vi "PI Terminal.vi"() -> ()   [LabVIEW 2013]
doc: "HELP for Terminal.vi\n\nThe terminal VI is a stand-alone application. It first asks the user to specify the full configuration (number of controlled systems, RS-232, GPIB, TCP-IP or DLL communication, communications parameters), then it establishes a connection with a selected system. This will work for all PI devices which support the PI General Command Set, or at least follow the same syntax rules and support the *IDN? and ERR? commands.\n\nAfter starting the VI, the interface parameters of the systems with which to communicate must be selected. For this reason, \"PITerminal.vi\" calls \"PI Ask for Communication Parameters.vi\". Select here the number of connected PI systems that you want to communicate with. For each system, select the appropriate interface parameters. \n\nC-702: Interface = RS232 or TCP/IP, RS232: Input and output HW handshake must be TRUE. Syntax: GCS 1.0; Term char = LF.\n\nC-843: Interface = DLL, DLL for Device = C-843, DLL Interface = Board, Parameter = Board number (1 for first C-843 board). Syntax: GCS 1.0; Term char = LF.\n\nC-843.PM: Interface = DLL, DLL for Device = C-843.PM, DLL Interface = Board, Parameter = Board number (1 for first C-843 board). Syntax: GCS 1.0; Term char = LF.\n\nC-844: Interface = DLL, DLL for Device = C-844, DLL Interface = RS232 or GPIB, Parameter = empty string, RS232 baud rate = 9600. Syntax: GCS 1.0; Term char = LF.\n\nC-865: Interface = DLL, DLL for Device = C-865, DLL Interface = RS232, Parameter = empty string, RS232 baud rate = set as appropriate. Syntax: GCS 1.0; Term char = LF.\n\nC-866: Interface = DLL, DLL for Device = C-866, DLL Interface = RS232 or USB, RS232: Parameter = empty string, RS232 baud rate = set as appropriate, USB: Parameter = Serial no. of system to connect to, Syntax: GCS 1.0; Term char = LF.\n\nC-867: Single Device: Interface = RS232 or DLL, RS232: Input and output HW handshake must be FALSE. DLL (USB): DLL for Device = C-867, DLL Interface = USB, Parameter = Serial no. of system to connect to. DaisyChain: Interface = DLL, DLL for Device = C-867, DLL Interface = RS232_DC, Parameter = Number of device in chain, Register DC: FALSE. Syntax: GCS 2.0; Term char = LF.\n\nC-880, C-848: Interface = RS232 or GPIB, RS232: Input and output HW handshake must be TRUE. Syntax: GCS 1.0; Term char = LF.\n\nC-880K005: Interface = RS232, Input and output HW handshake must be FALSE. Syntax: GCS 1.0; Term char = LF.\n\nE-516: Interface = RS232 or GPIB, RS232: Input and output HW handshake must be TRUE. Syntax: GCS 1.0; Term char = LF.\n\nE-517: Interface = RS232, GPIB, TCP/IP or DLL, RS232: Input and output HW handshake must be TRUE, DLL (USB): DLL for Device = E-517, DLL Interface = USB, Parameter = Serial no. of system to connect to. Syntax: GCS 2.0; Term char = LF.\n\nE-709: Interface = RS232 or DLL, RS232: Input and output HW handshake must be TRUE. DLL (USB): DLL for Device = E-709, DLL Interface = USB, Parameter = Serial no. of system to connect to. Syntax: GCS 2.0; Term char = LF.\n\nE-710: Interface = DLL, DLL for Device = E-710, DLL Interface = RS232 or GPIB, Parameter = empty string. Syntax: GCS 1.0; Term char = LF.\n\nE-712: Interface = RS232, TCP/IP or DLL, RS232: Input and output HW handshake must be TRUE. DLL: DLL for Device = E-712, DLL Interface = USB, Parameter = Serial no. of system to connect to. Syntax: GCS 2.0; Term char = LF.\n\nE-725: Interface = RS232, TCP/IP or DLL, RS232: Input and output HW handshake must be TRUE. DLL: DLL for Device = E-725, DLL Interface = USB, Parameter = Serial no. of system to connect to. Syntax: GCS 2.0; Term char = LF.\n\nE-753: Interface = RS232 or TCP/IP, RS232: Input and output HW handshake must be TRUE. Syntax: GCS 2.0; Term char = LF.\n\nE-755: Single Device: Interface = RS232, Input and output HW handshake must be TRUE. DaisyChain: Interface = DLL, DLL for Device = E-755, DLL Interface = RS232_DC, Parameter = Number of device in chain (first device: 1). Syntax: GCS 2.0; Term char = LF.\n\nE-761: Interface = DLL, DLL for Device = E-761, DLL Interface = Board, Parameter = Board number (1 for first E-761 board). Syntax: GCS 1.0; Term char = LF.\n\nE-816: Interface = RS232 or DLL, RS232: Input and output HW handshake must be TRUE. DLL (USB): DLL for Device = E-816, DLL Interface = USB, Parameter = Serial no. of system to connect to. Syntax: GCS 1.0; Term char = LF. \n\nE-861: Single Device: Interface = RS232 or DLL, RS232: Input and output HW handshake must be FALSE. DLL (USB): DLL for Device = E-861, DLL Interface = USB, Parameter = Serial no. of system to connect to. DaisyChain: Interface = DLL, DLL for Device = E-861, DLL Interface = RS232_DC, Parameter = Number of device in chain (first device: 1), Register DC: FALSE. Syntax: GCS 2.0; Term char = LF.\n\nF-206, M-8X0: For GCS syntax version = GCS 1.0 (older firmware or compatibility mode, can be set with CSV.vi), Interface = RS232, GPIB (not available for C-887 controller) or TCP/IP., The error status will not be cleared by this VI. The first ERR? query will report a hidden error with error code 1, which will be cleared during system initialization (INI). RS232: Input and output handshake settings must be FALSE. Syntax: GCS 1.0; Term char = LF.\n For GCS syntax version = GCS 2.0 (C-887 Controller), Interface = RS232 or TCP/IP. RS232: Input and output handshake settings must be FALSE. Syntax: GCS 2.0; Term char = LF.\n\nMercury™: Interface = DLL, DLL for Device = Mercury™, DLL Interface = RS232 (even if using USB), Parameter = empty string, RS232 baud rate = same as set on controller hardware. Syntax: GCS 1.0; Term char = LF.\n\nGCS_Mercury: Single Device: Interface = RS232 or DLL, RS232: Input and output HW handshake must be FALSE. DLL (USB): DLL for Device = PI_GCS2_DLL, DLL Interface = USB, Parameter = Serial no. of system to connect to.\n DaisyChain: Interface = DLL, DLL for Device = PI_GCS2_DLL, DLL Interface = RS232_DC, Parameter = Number of device in chain, Register DC: FALSE. Syntax: GCS 2.0; Term char = LF.\n\nIf the chosen timeout value is greater than 1000 ms, it will automatically be set to 1000 ms for a fluid program operation. \n\nIn the upper window (\"Send\") the user can enter commands which will be transmitted to the chosen device one line at a time when the ENTER key is pressed. \nAll controller responses are displayed in the Receive response window, which can be cleared by pressing the Clear Receive Window button or F2. \n\nThe view style of the Receive window can be changed to Show all characters or Hex View using the menu ring above the Receive window.\n\nExit or F10 will terminate the terminal application. \n\nTo send the last command again, just press the ENTER key again. The next line will then show the following entry: \"(Send: cmd)\" with cmd being the command from the line before, which was resent.\n\nWhen the terminal application has just been started, pressing ENTER without entering a command will send \"*IDN?\" to the chosen system. \n\nNew commands can only be inserted into the last line of the Send window. The user can scroll through the history of the Send window using the scroll bar or the cursor up/down keys, but cannot change the history or resend commands by pressing ENTER unless in the last line. Pressing ENTER will always resend the last command, no matter where the cursor is positioned. Selecting text and using copy and paste (Ctrl+C, Ctrl+V) works for single lines, if only the contents of one single line (the command text) is selected and copied, not the full line (including the LineFeed) or multiple lines.\n\nMany of PI's General Command Set compatible devices support single-byte commands. For example, the user can stop a fast scan of a C-880 or F-206 by sending an ASCII 24 (decimal). To enter this command into the Send window simply type a \"#\" followed by the decimal value of the byte to be sent, e.g. enter \"#24\" and presses ENTER to stop a fast scan. An entry \"(Send: *)\" will be added to the original command with * being the corresponding ASCII character of the single byte sent. \n\nPressing F1 or the Help button will pop up a help window. To return to the terminal application, press Esc. If Send ERR? on Exit? is TRUE, an \"ERR?\" query is sent to the device when Exit is pressed to prevent the controller from keeping an error condition produced during the use of the terminal application."
uses:
  Low Level/Communication.llb/Available DLLs.ctl
  Low Level/Communication.llb/Termination character.ctl
panel:
  in  "HowTo":string="Start application and choose interface parameters in next window."
  out "TCP/IP Config. System":T1={"Host address/name"="Z-A521-2.pi.ws", "Port"=3000, "Board"=0, "Timeout"=5000}
  out "Help string":string="\nHELP for Terminal.vi\n\nThis terminal application works for all PI devices which support the PI General Command Set or at least follow the syntax rules of this command structure and support the commands *IDN? and ERR?.\n\nIn the upper window (\"Send\") the user can enter commands which will be transmitted to the chosen device one line at a time when the ENTER key is pressed. All controller responses are displayed in the Receive response window, which can be cleared by pressing the Clear Receive Window button or F2. The view style of the Receive window can be changed to Show all characters or Hex View using the menu ring above the Receive window.\n\nExit or F10 will terminate the terminal application. \n\nTo send the last command again, just press the ENTER key again. The next line will then show the following entry: \"(Send: cmd)\" with cmd being the command from the line before, which was resent.\nWhen the terminal application has just been started, pressing ENTER without entering a command will send \"*IDN?\" to the chosen system.\n\nNew commands can only be inserted into the last line of the Send window. The user can scroll through the history of the Send window using the scroll bar or the cursor up/down keys, but cannot change the history or resend commands by pressing ENTER unless in the last line. Pressing ENTER will always resend the last command, no matter where the cursor is positioned. Selecting text and using copy and paste (Ctrl+C, Ctrl+V) works for single lines, if only the contents of one single line (the command text) is selected and copied, not the full line (including the LineFeed) or multiple lines.\n\nMany of PI's General Command Set compatible devices support single-byte commands. For example, the user can stop a fast scan of a C-880 or F-206 by sending an ASCII 24 (decimal). To enter this command into the Send window simply type a \"#\" followed by the decimal value of the byte to be sent, e.g. enter \"#24\" and presses ENTER to stop a fast scan. An entry \"(Send: *)\" will be added to the original command with * being the corresponding ASCII character of the single byte sent. \n\nIf Send ERR? on Exit? is TRUE, a \"ERR?\" query is sent to the device when Exit is pressed to prevent the controller from keeping an error condition produced during the use of the terminal application.\n\nC-702: \tInterface = RS232 or TCP/IP, RS232: Input and output HW handshake \tmust \tbe TRUE. Syntax: GCS 1.0; Term char = LF.\n\nC-843: \tInterface = DLL, DLL for Device = C-843, DLL Interface = Board, \tParameter = Board number (1 for first C-843 board). Syntax: GCS 1.0; \tTerm char = LF.\n\nC-843.PM: \tInterface = DLL, DLL for Device = C-843.PM, DLL Interface = Board, \tParameter = Board number (1 for first C-843 board). Syntax: GCS 1.0; \tTerm char = LF.\n\nC-865: \tInterface = DLL, DLL for Device = C-865, DLL Interface = RS232, \tParameter = empty string, RS232 baud rate = set as appropriate. Syntax: \tGCS 1.0; Term char = LF.\n\nC-866: \tInterface = DLL, DLL for Device = C-866, DLL Interface = RS232 or USB, \tRS232: Parameter = empty string, RS232 baud rate = set as appropriate, \tUSB: Parameter = Serial no. of system to connect to, \n\tSyntax: GCS 1.0; Term char = LF.\n\nC-867: \tSingle Device: Interface = RS232 or DLL, RS232: Input and output HW \thandshake must be FALSE. DLL (USB): DLL for Device = C-867, DLL \tInterface = USB, Parameter = Serial no. of system to connect to.\nDaisyChain: Interface = DLL, DLL for Device = C-867, DLL Interface = \tRS232_DC, Parameter = Number of device in chain, \tRegister DC: \tFALSE. Syntax: GCS 2.0; Term char = LF.\n\nC-880, C-848: \tInterface = RS232 or GPIB, RS232: Input and output HW handshake must \tbe TRUE. Syntax: GCS 1.0; Term char = LF.\n\nC-880K005: \tInterface = RS232, Input and output HW handshake must be FALSE. \tSyntax: GCS 1.0; Term char = LF.\n\nE-516: \tInterface = RS232 or GPIB, RS232: Input and output HW handshake must \tbe TRUE. Syntax: GCS 1.0; Term char = LF.\n\nE-517: \tInterface = RS232, GPIB, TCP/IP or DLL, RS232: Input and output HW \thandshake must be TRUE, DLL (USB): DLL for Device = E-517, DLL \tInterface = USB, Parameter = Serial no. of system to connect to. \nSyntax: GCS 2.0; Term char = LF.\n\nE-709: \tInterface = RS232 or DLL, RS232: Input and output HW handshake \tmust be TRUE. DLL (USB): DLL for Device = E-709, DLL Interface = USB, \tParameter = Serial no. of system to connect to. Syntax: GCS 2.0; Term \tchar = LF.\n\nE-710:\tInterface = DLL, DLL for Device = E-710, DLL Interface = RS232 or GPIB, \tParameter = empty string. Syntax: GCS 1.0; Term char = LF.\n\nE-712: \tInterface = RS232, TCP/IP or DLL, RS232: Input and output HW \thandshake must be TRUE. DLL: DLL for Device = E-712, DLL Interface = \tUSB, \tParameter = Serial no. of system to connect to. \n\tSyntax: GCS 2.0; Term char = LF.\n\nE-725: \tInterface = RS232, TCP/IP or DLL, RS232: Input and output HW \thandshake must be TRUE. DLL: DLL for Device = E-725, DLL Interface = \tUSB, \tParameter = Serial no. of system to connect to. \nSyntax: GCS 2.0; Term char = LF.\n\nE-753: \tInterface = RS232 or TCP/IP, RS232: Input and output HW handshake \tmust \tbe TRUE. Syntax: GCS 2.0; Term char = LF.\n\nE-755:\tSingle Device: Interface = RS232, Input and output HW handshake must \tbe TRUE. DaisyChain: Interface = DLL, DLL for Device = E-755, DLL \tInterface = RS232_DC, Parameter = Number of device in chain (first \tdevice: 1). Syntax: GCS 2.0; Term char = LF.\n\nE-761:\tInterface = DLL, DLL for Device = E-761, DLL Interface = Board, \tParameter = Board number (1 for first E-761 board). Syntax: GCS 1.0; \tTerm char = LF.\n\nE-816: \tInterface = RS232 or DLL, RS232: Input and output HW handshake must \tbe TRUE. DLL (USB): DLL for Device = E-816, DLL Interface = USB, \tParameter = Serial no. of system to connect to. Syntax: GCS 1.0; Term \tchar = LF. \n\nE-861: \tSingle Device: Interface = RS232 or DLL, RS232: Input and output HW \thandshake must be FALSE. DLL (USB): DLL for Device = E-861, DLL \tInterface = USB, Parameter = Serial no. of system to connect to.\nDaisyChain: Interface = DLL, DLL for Device = E-861, DLL Interface = \tRS232_DC or USB_DC, Parameter = Number of device in chain (first device: 1), \tRegister DC: FALSE. Syntax: GCS 2.0; Term char = LF.\n\nF-206, M-8X0: \tFor GCS syntax version = GCS 1.0 (older firmware or compatibility mode, \tcan be set with CSV.vi), Interface = RS232, GPIB (not available for C-887 \tcontroller) or TCP/IP., The error status will not be cleared by this VI. The \tfirst ERR? query will report a hidden error with error code 1, which will be \tcleared during system initialization (INI). RS232: Input and output \thandshake settings must be FALSE. Syntax: GCS 1.0; Term char = \tLF.\n\tFor GCS syntax version = GCS 2.0 (C-887 Controller), Interface = RS232 \tor TCP/IP. RS232: Input and output handshake settings must be FALSE. \tSyntax: GCS 2.0; Term char = LF.\n\nMercury™: \tInterface = DLL, DLL for Device = Mercury™, DLL Interface = RS232 \t(even if using USB), Parameter = empty string, RS232 baud rate = same \tas set on controller hardware, Syntax: GCS 1.0; Term char = LF.\n\nGCS_Mercury: \tSingle Device: Interface = RS232 or DLL, RS232: Input and output HW \thandshake must be FALSE. DLL (USB): DLL for Device = PI_GCS2_DLL, \tDLL Interface = USB, Parameter = Serial no. of system to connect to. \tDaisyChain: Interface = DLL, DLL for Device = PI_GCS2_DLL, DLL \tInterface = RS232_DC or USB_DaisyChain, Parameter = Number of device in chain, \tRegister DC: \tFALSE. Syntax: GCS 2.0; Term char = LF.\n\nPress Esc to return to the terminal application."
  in  "ERR? on exit?":bool=TRUE
  out "error out":T2
  out "GPIB Configuration system":T3={"bus"=0, "address"=4, "mode"=0, "Timeout"=1000}
  out "DLL for Device":T4 items=["C-843", "C-844", "E-710", "C-843.PM", "C-865", "E-761", "Mercury", "E-755", "E-753", "C-866", "E-712", "E-725", "E-861", "C-867", "E-517", "E-816", "E-709", "PI_GCS2_DLL"]
  in  "Hide help":bool
  in  "Show help":bool
  in  "View style":u16(ring) items=["Normal view", "Show all characters", "Hex View"]
  out "error":bool
  in  "Send":bool
  in  "Clear":bool
  in  "Exit":bool
  out "Receive":string
  in  "System No.":i32=1 min=1 step=1
  out "Interface":u16(ring) items=["RS232", "GPIB", "DLL", "TCP/IP"]
  out "System ind.":i32=1
  out "System":i32=1
  out "RS232 Config. System":T5={"RS232 Portnumber"=0, "Timeout"=1000, "Baudrate"=57600, "Handshake"=0} {"Handshake" items=["None", "HW", "XON/XOFF"]; "RS232 Portnumber" items=["COM1", "COM2", "COM3", "COM4", "COM5", "COM6", "COM7", "COM8", "COM9", "COM10", "COM11", "COM12", "COM13", "COM14", "COM15", "COM16", "COM17", "COM18", "COM19", "COM20", "COM21", "COM22", "COM23", "COM24", "COM25", "COM26", "COM27", "COM28", "COM29", "COM30"]}
  in  "Send":string="*IDN?\n"
  out "Term.char":T6
  # "Terminal"
  # "If chosen timeout value is > 1000 ms, \nit will be set to 300 ms."
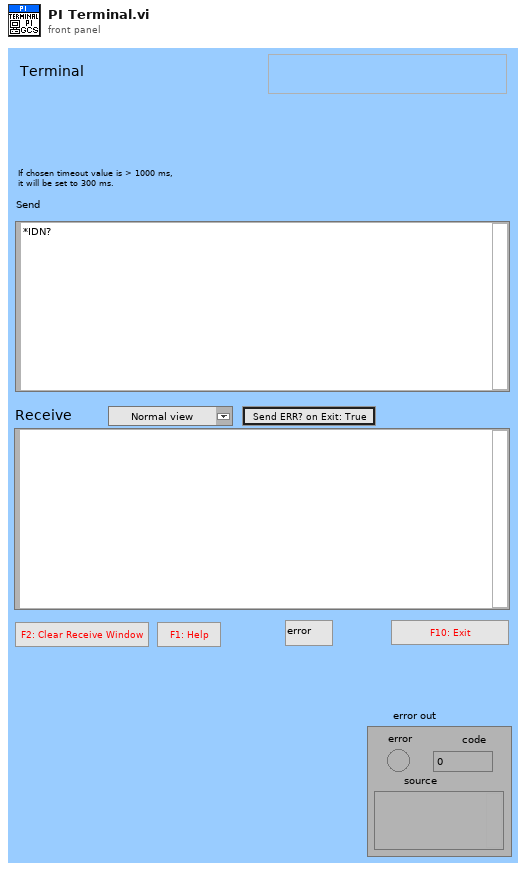
[diagram p1: front panel]
types:
  T1 = cluster{"Host address/name":string, "Port":i32, "Board":i32, "Timeout":i32}
  T2 = cluster{"error":bool, "code":i32, "source":string}
  T3 = cluster{"bus":i16, "address":i16, "mode":i16, "Timeout":i32}
  T4 = typedef "Available DLLs.ctl" = u16
  T5 = cluster{"RS232 Portnumber":i32, "Timeout":i32, "Baudrate":u32, "Handshake":u16}
  T6 = typedef "Termination character.ctl" = enum16{"LF", "CR", "LFCR", "CRLF"}
  T7 = cluster{"data bits":u16, "stop bits":enum16{"1 bit", "1.5 bits", "2 bits"}, "parity":enum16{"no parity", "odd parity", "even parity", "mark parity", "space parity"}}
  T8 = cluster{"Host address/name":string, "Port":i32, "Board":i32}[]
  T9 = cluster{"input XON/XOFF":bool, "input HW Handshake":bool, "input alt HW HShk":bool, "output XON/XOFF":bool, "output HW Handshake":bool, "output alt HW HShk":bool, "XOFF byte ":u8, "XON byte":u8, "parity error byte":u16}[]
  T10 = typedef "Available interfaces.ctl" = u16
  T11 = cluster{"RS232 Portnumber":u16, "Timeout":u32, "RS232 baud rate":u32, "Interface":T10, "GPIB Bus":i16, "GPIB address":i16, "GPIB Mode":i16}[]
  T12 = typedef "Available DLL interfaces.ctl" = u16
  T13 = cluster{"DLL for Device":T4, "DLL Interface":T12, "Parameter":string}[]
  T14 = cluster{"RS232 Portnumber":u16, "Timeout":u32, "RS232 baud rate":u32, "Interface":T10, "GPIB Bus":i16, "GPIB address":i16, "GPIB Mode":i16}
  T15 = cluster{"Portnumber":u32, "Timeout":i32, "Baudrate":u32, "Handshake":u16}
  T16 = cluster{"data bits":u16, "stop bits":enum16{"1 bit", "1.5 bits", "2 bits"}, "parity":enum16{"no parity", "odd parity", "even parity", "mark parity", "space parity"}}[]
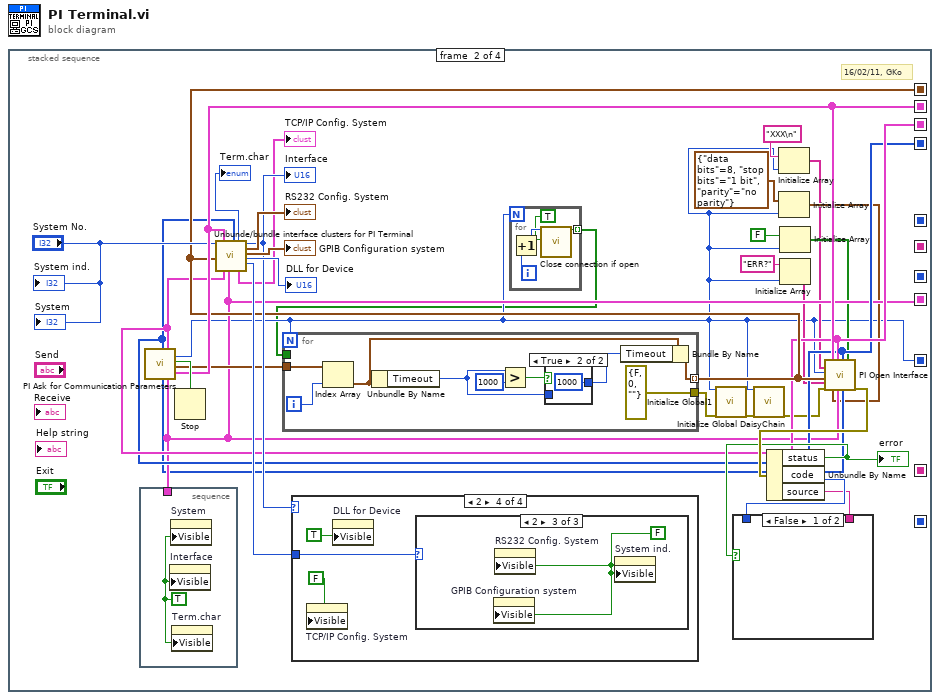
[diagram p0: block diagram]
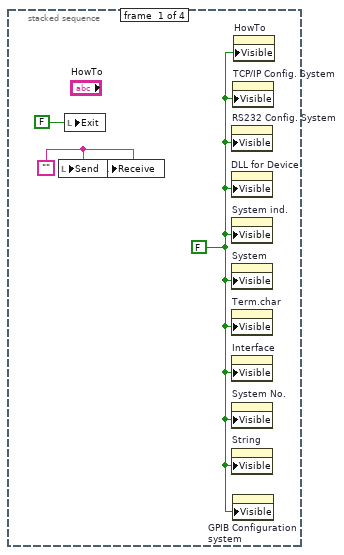
[diagram p2: hidden frame]
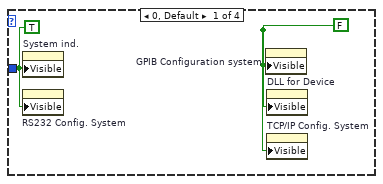
[diagram p3: hidden frame]
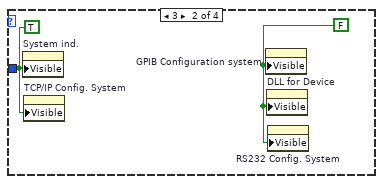
[diagram p4: hidden frame]
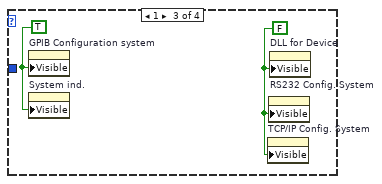
[diagram p5: hidden frame]
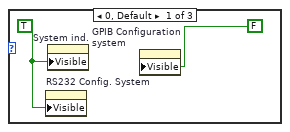
[diagram p6: hidden frame]
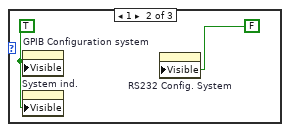
[diagram p7: hidden frame]
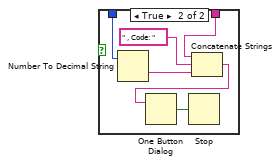
[diagram p8: hidden frame]
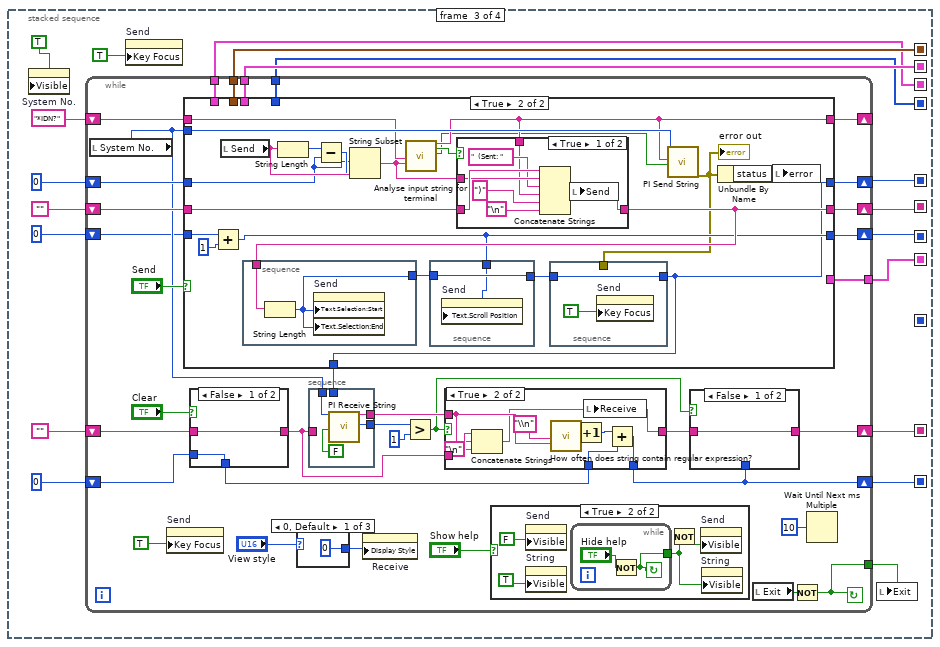
[diagram p10: hidden frame]
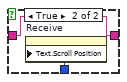
[diagram p12: hidden frame]
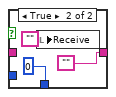
[diagram p13: hidden frame]
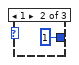
[diagram p15: hidden frame]
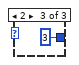
[diagram p16: hidden frame]
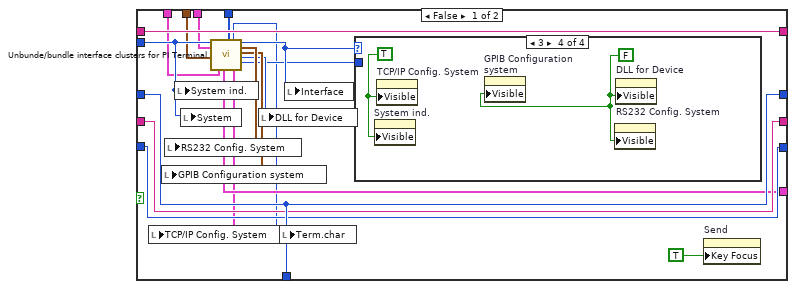
[diagram p17: hidden frame]
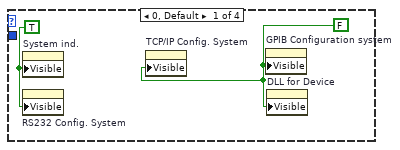
[diagram p18: hidden frame]
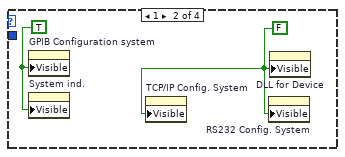
[diagram p19: hidden frame]
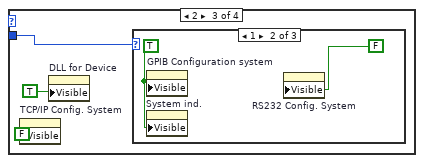
[diagram p20: hidden frame]
diagram:
  n1 = stacked-sequence {
    seq-local: [_ w23 _ _] -> [_ _ w90 _]
    seq-local: [_ w32 _ _] -> [_ _ w89 _]
    seq-local: [_ w18 _ _] -> [_ _ w80 _]
    seq-local: [_ _ w79 _] -> [_ _ _ w232]
    seq-local: [_ _ w78 _] -> [_ _ _ w231]
    seq-local: [_ _ w77 _] -> [_ _ _ w233]
    seq-local: [_ _ w76 _] -> [_ _ _ w234]
    seq-local: [_ _ w75 _] -> [_ _ _ w235]
    seq-local: [_ w20 _ _] -> [_ _ w74 _]
    seq-local: [_ w19 _ _] -> [_ _ w73 _]
    seq-local: [_ w6 _ _] -> [_ _ _ w229]
    frame #0 {
      w1 = FALSE ("Visible")
      w3 = ""
      n2 = local write "Send"(w3) -> ()
      n3 = local write "Exit"(FALSE ("error")) -> ()
      n4 = local write "Receive"(w3) -> ()
      n5 = property on="RS232 Config. System" class="Clust (strict)"("Visible"=w1) -> ()  [unwired: 2 in, 2 out]
      n6 = property on="DLL for Device" class="Ring (strict)"("Visible"=w1) -> ()  [unwired: 2 in, 2 out]
      n7 = property on="System ind." class="DigNum (strict)"("Visible"=w1) -> ()  [unwired: 2 in, 2 out]
      n8 = property on="System" class="DigNum (strict)"("Visible"=w1) -> ()  [unwired: 2 in, 2 out]
      n9 = property on="Term.char" class="Enum (strict)"("Visible"=w1) -> ()  [unwired: 2 in, 2 out]
      n10 = property on="Interface" class="Ring (strict)"("Visible"=w1) -> ()  [unwired: 2 in, 2 out]
      n11 = property on="System No." class="DigNum (strict)"("Visible"=w1) -> ()  [unwired: 2 in, 2 out]
      n12 = property on="String" class="Str"("Visible"=w1) -> ()  [unwired: 2 in, 2 out]
      n13 = property on="TCP/IP Config. System" class="Clust (strict)"("Visible"=w1) -> ()  [unwired: 2 in, 2 out]
      n14 = property on="GPIB Configuration system" class="Clust (strict)"("Visible"=w1) -> ()  [unwired: 2 in, 2 out]
      n15 = property on="HowTo" class="Str"("Visible"=w1) -> ()  [unwired: 2 in, 2 out]
    }
    frame #1 {
      # "16/02/11, GKo"
      n16 = call "PI Ask for Communication Parameters.vi"() -> ("Termination character out"=w19:T6[], "Syntax out"=w17:enum16{"GCS 1.0", "GCS 2.0"}[], "TCP/IP Configuration out"=w20:T8, "Flow control out"=w18:T9, "How many\nsystems? out"=w6:i32, "Abort out"=w35:bool, "Interface configuration out"=w24:T11, "DLL Interface\nconfiguration out"=w32:T13)  [unwired: 12 out]
      n17 = stacked-sequence {
        tunnel: w18 -> [_]
        frame #0 {
          w41 = TRUE ("Visible")
          n18 = property on="Interface" class="Ring (strict)"("Visible"=w41) -> ()  [unwired: 2 in, 2 out]
          n19 = property on="System" class="DigNum (strict)"("Visible"=w41) -> ()  [unwired: 2 in, 2 out]
          n20 = property on="Term.char" class="Enum (strict)"("Visible"=w41) -> ()  [unwired: 2 in, 2 out]
        }
      }
      n21 = Stop(stop? (T)=w35) -> ()
      n22 = for {
        N: w6 -> [_]
        tunnel: [w37] -> w5 mode=indexing
        i -> [w40]
        n23 = Increment(x=w40) -> (x+1=w39:i32)
        n24 = call "Close connection if open.vi"("System no."=w39, "Close DaisyChain"=TRUE) -> ("Was connected?"=w37:bool)  [unwired: 1 in, 16 out]
      }
      n25 = for {
        N: w6 -> [_]
        tunnel: w24 -> [w69]
        tunnel: [w68] -> w23 mode=indexing
        tunnel: w5 -> [_]
        tunnel: [errorcluster {"status"=FALSE, "code"=0, "source"=""} ("error in")] -> w4
        i -> [w70]
        n26 = Index Array(array=w69, index=w70) -> (element=w65:T14)
        n27 = Unbundle By Name(w65) -> ("Timeout"=w64:u32)
        n28 = Greater?(x=w64, y=u32 1000) -> (0:w63:bool)
        n29 = case shown="True" w63 {
          tunnel: [w71 1000] -> w66
          tunnel: w64 -> [w71 _]
          frame False {
          }
          frame True {
          }
        }
        n30 = Bundle By Name(cluster=w65, "Timeout"=w66) -> (w68:T14)
      }
      n31 = call "Unbunde/bundle interface clusters for PI Terminal.vi"("System No."="System No.", "Interface configuration"=w23, "DLL Interface\nconfiguration"=w32, "TCP/IP Configuration"=w20, "Flow control"=w18, "Termination character"=w19) -> ("Term.char"=→"Term.char":T6, "TCP/IP Config. System"=→"TCP/IP Config. System":T1, "Interface"=w27:T10, "RS232 configuration system"=→"RS232 Config. System":T15, "GPIB configuration system"=→"GPIB Configuration system":T3, "DLL for device"=→"DLL for Device":T4, "DLL interface"=w26:T12)  [unwired: 7 out]
      "Interface" <- w27
      n32 = case shown="2" w27 {
        tunnel: w26 -> [_ _ _ w49]
        frame 0, Default {
          w42 = FALSE ("Write Attribute")
          w43 = TRUE ("Write Attribute")
          n33 = property on="System ind." class="DigNum (strict)"("Visible"=w43) -> ()  [unwired: 2 in, 2 out]
          n34 = property on="RS232 Config. System" class="Clust (strict)"("Visible"=w43) -> ()  [unwired: 2 in, 2 out]
          n35 = property on="GPIB Configuration system" class="Clust (strict)"("Visible"=w42) -> ()  [unwired: 2 in, 2 out]
          n36 = property on="DLL for Device" class="Ring (strict)"("Visible"=w42) -> ()  [unwired: 2 in, 2 out]
          n37 = property on="TCP/IP Config. System" class="Clust (strict)"("Visible"=w42) -> ()  [unwired: 2 in, 2 out]
        }
        frame 3 {
          w45 = FALSE ("Write Attribute")
          w44 = TRUE ("Write Attribute")
          n38 = property on="System ind." class="DigNum (strict)"("Visible"=w44) -> ()  [unwired: 2 in, 2 out]
          n39 = property on="TCP/IP Config. System" class="Clust (strict)"("Visible"=w44) -> ()  [unwired: 2 in, 2 out]
          n40 = property on="GPIB Configuration system" class="Clust (strict)"("Visible"=w45) -> ()  [unwired: 2 in, 2 out]
          n41 = property on="DLL for Device" class="Ring (strict)"("Visible"=w45) -> ()  [unwired: 2 in, 2 out]
          n42 = property on="RS232 Config. System" class="Clust (strict)"("Visible"=w45) -> ()  [unwired: 2 in, 2 out]
        }
        frame 1 {
          w47 = TRUE ("Write Attribute")
          w46 = FALSE ("Write Attribute")
          n43 = property on="GPIB Configuration system" class="Clust (strict)"("Visible"=w47) -> ()  [unwired: 2 in, 2 out]
          n44 = property on="System ind." class="DigNum (strict)"("Visible"=w47) -> ()  [unwired: 2 in, 2 out]
          n45 = property on="TCP/IP Config. System" class="Clust (strict)"("Visible"=w46) -> ()  [unwired: 2 in, 2 out]
          n46 = property on="RS232 Config. System" class="Clust (strict)"("Visible"=w46) -> ()  [unwired: 2 in, 2 out]
          n47 = property on="DLL for Device" class="Ring (strict)"("Visible"=w46) -> ()  [unwired: 2 in, 2 out]
        }
        frame 2 {
          n48 = property on="TCP/IP Config. System" class="Clust (strict)"("Visible"=FALSE) -> ()  [unwired: 2 in, 2 out]
          n49 = property on="DLL for Device" class="Ring (strict)"("Visible"=TRUE ("Write Attribute")) -> ()  [unwired: 2 in, 2 out]
          n50 = case shown="2" w49 {
            frame 0, Default {
              w51 = TRUE ("Write Attribute")
              n51 = property on="RS232 Config. System" class="Clust (strict)"("Visible"=w51) -> ()  [unwired: 2 in, 2 out]
              n52 = property on="System ind." class="DigNum (strict)"("Visible"=w51) -> ()  [unwired: 2 in, 2 out]
              n53 = property on="GPIB Configuration system" class="Clust (strict)"("Visible"=FALSE ("Write Attribute")) -> ()  [unwired: 2 in, 2 out]
            }
            frame 1 {
              w53 = TRUE ("Write Attribute")
              n54 = property on="GPIB Configuration system" class="Clust (strict)"("Visible"=w53) -> ()  [unwired: 2 in, 2 out]
              n55 = property on="System ind." class="DigNum (strict)"("Visible"=w53) -> ()  [unwired: 2 in, 2 out]
              n56 = property on="RS232 Config. System" class="Clust (strict)"("Visible"=FALSE ("Write Attribute")) -> ()  [unwired: 2 in, 2 out]
            }
            frame 2 {
              w55 = FALSE ("Write Attribute")
              n57 = property on="GPIB Configuration system" class="Clust (strict)"("Visible"=w55) -> ()  [unwired: 2 in, 2 out]
              n58 = property on="RS232 Config. System" class="Clust (strict)"("Visible"=w55) -> ()  [unwired: 2 in, 2 out]
              n59 = property on="System ind." class="DigNum (strict)"("Visible"=w55) -> ()  [unwired: 2 in, 2 out]
            }
          }
        }
      }
      n60 = call "Initialize Global1.vi"("System no."=w6, "error in"=w4) -> ("error out"=w16:errorcluster)  [unwired: 17 out]
      n61 = call "Initialize Global DaisyChain.vi"("System no."=w6, "error in"=w16) -> ("error out"=w15:errorcluster)  [unwired: 17 out]
      n62 = Initialize Array("XXX\n", w6) -> (w8:string[])
      n63 = Initialize Array(T7 {"data bits"=8, "stop bits"=enum."1 bit", "parity"=enum."no parity"} ("Bit settings and parity"), w6) -> (w10:T16)
      n64 = Initialize Array(FALSE ("Register DC"), w6) -> (w14:bool[])
      n65 = Initialize Array("ERR?", w6) -> (w12:string[])
      n66 = call "PI Open Interface.vi"("Interface clear"=w8, "Number of systems"=w6, "Interface configuration"=w23, "Strings to send"=w12, "error in"=w15, "DLL Interface\nConfiguration"=w32, "Bit settings and parity"=w10, "TCP/IP\nConfiguration"=w20, "Flow control"=w18, "Termination character"=w19, "Syntax"=w17, "Register DC"=w14) -> ("error out"=w36:errorcluster)  [unwired: 7 out]
      n67 = Unbundle By Name(w36) -> ("status"=w25:bool, "code"=w34:i32, "source"=w33:string)
      "error" <- w25
      n68 = case shown="False" w25 {
        tunnel: w34 -> [_ w60]
        tunnel: w33 -> [_ w59]
        frame False {
        }
        frame True {
          n69 = Number To Decimal String(number=w60) -> (decimal integer string=w57:string)  [unwired: 1 out]
          n70 = Concatenate Strings(w59, " , Code: " ("Substring"), w57) -> (w56:string)
          n71 = One Button Dialog(message=w56) -> (true=w61:bool)  [unwired: 1 out]
          n72 = Stop(stop? (T)=w61) -> ()
        }
      }
      "System ind." <- "System No."
      "System" <- "System No."
    }
    frame #2 {
      n73 = property on="System No." class="DigNum (strict)"("Visible"=TRUE ("Write Attribute")) -> ()  [unwired: 2 in, 2 out]
      n74 = while {
        tunnel: w80 -> [w95]
        tunnel: [w96] -> w81
        shift-left: 0 -> [w109]
        shift-right: [w108] -> w77
        shift-left: 0 -> [w105]
        shift-right: [w99] -> w78
        shift-left: "" -> [w106]
        shift-right: [w100] -> w79
        shift-left: "" -> [w117]
        shift-right: [w116] -> w76
        shift-left: 0 -> [w121]
        shift-right: [w120] -> w75
        tunnel: w89 -> [w125]
        tunnel: w90 -> [w126]
        shift-left: "*IDN?" -> [w123]
        shift-right: [w122] -> _
        tunnel: w74 -> [w93]
        tunnel: w73 -> [w92]
        stop <- w96 continue-if-true
        n75 = local read "System No."() -> (w114:i32)
        n76 = property on="Send" class="Str"("Key Focus"=TRUE ("Write Attribute")) -> ()  [unwired: 2 in, 2 out]
        n77 = case shown="True" "Send" {
          tunnel: w114 -> [w171 w210]
          tunnel: w126 -> [w170 _]
          tunnel: w125 -> [w169 _]
          tunnel: w123 -> [w176 w208]
          tunnel: [w176 w205] -> w122
          tunnel: w121 -> [w175 w196]
          tunnel: [w175 w193] -> w120
          tunnel: w117 -> [w172 w204]
          tunnel: [w172 w200] -> w116
          tunnel: [w175 w193] -> w115
          tunnel: w109 -> [w173 w199]
          tunnel: [w173 w195] -> w108
          tunnel: w95 -> [w163 _]
          tunnel: w93 -> [w162 _]
          tunnel: w92 -> [w161 _]
          frame False {
            n78 = local write "System ind."(w171) -> ()
            n79 = local write "System"(w171) -> ()
            n80 = call "Unbunde/bundle interface clusters for PI Terminal.vi"("System No."=w171, "Interface configuration"=w170, "DLL Interface\nconfiguration"=w169, "TCP/IP Configuration"=w162, "Flow control"=w163, "Termination character"=w161) -> ("Term.char"=w159:T6, "TCP/IP Config. System"=w160:T1, "Interface"=w165:T10, "RS232 configuration system"=w168:T15, "GPIB configuration system"=w167:T3, "DLL for device"=w166:T4, "DLL interface"=w164:T12)  [unwired: 7 out]
            n81 = local write "TCP/IP Config. System"(w160) -> ()
            n82 = local write "GPIB Configuration system"(w167) -> ()
            n83 = local write "RS232 Config. System"(w168) -> ()
            n84 = local write "DLL for Device"(w166) -> ()
            n85 = local write "Term.char"(w159) -> ()
            n86 = local write "Interface"(w165) -> ()
            n87 = case shown="3" w165 {
              tunnel: w164 -> [_ _ w182 _]
              frame 0, Default {
                w177 = FALSE ("Write Attribute")
                w178 = TRUE ("Write Attribute")
                n88 = property on="System ind." class="DigNum (strict)"("Visible"=w178) -> ()  [unwired: 2 in, 2 out]
                n89 = property on="RS232 Config. System" class="Clust (strict)"("Visible"=w178) -> ()  [unwired: 2 in, 2 out]
                n90 = property on="TCP/IP Config. System" class="Clust (strict)"("Visible"=w177) -> ()  [unwired: 2 in, 2 out]
                n91 = property on="GPIB Configuration system" class="Clust (strict)"("Visible"=w177) -> ()  [unwired: 2 in, 2 out]
                n92 = property on="DLL for Device" class="Ring (strict)"("Visible"=w177) -> ()  [unwired: 2 in, 2 out]
              }
              frame 1 {
                w180 = TRUE ("Write Attribute")
                w179 = FALSE ("Write Attribute")
                n93 = property on="GPIB Configuration system" class="Clust (strict)"("Visible"=w180) -> ()  [unwired: 2 in, 2 out]
                n94 = property on="System ind." class="DigNum (strict)"("Visible"=w180) -> ()  [unwired: 2 in, 2 out]
                n95 = property on="TCP/IP Config. System" class="Clust (strict)"("Visible"=w179) -> ()  [unwired: 2 in, 2 out]
                n96 = property on="RS232 Config. System" class="Clust (strict)"("Visible"=w179) -> ()  [unwired: 2 in, 2 out]
                n97 = property on="DLL for Device" class="Ring (strict)"("Visible"=w179) -> ()  [unwired: 2 in, 2 out]
              }
              frame 2 {
                n98 = property on="TCP/IP Config. System" class="Clust (strict)"("Visible"=FALSE) -> ()  [unwired: 2 in, 2 out]
                n99 = property on="DLL for Device" class="Ring (strict)"("Visible"=TRUE ("Write Attribute")) -> ()  [unwired: 2 in, 2 out]
                n100 = case shown="1" w182 {
                  frame 0, Default {
                    w184 = TRUE ("Write Attribute")
                    n101 = property on="RS232 Config. System" class="Clust (strict)"("Visible"=w184) -> ()  [unwired: 2 in, 2 out]
                    n102 = property on="System ind." class="DigNum (strict)"("Visible"=w184) -> ()  [unwired: 2 in, 2 out]
                    n103 = property on="GPIB Configuration system" class="Clust (strict)"("Visible"=FALSE ("Write Attribute")) -> ()  [unwired: 2 in, 2 out]
                  }
                  frame 1 {
                    w186 = TRUE ("Write Attribute")
                    n104 = property on="GPIB Configuration system" class="Clust (strict)"("Visible"=w186) -> ()  [unwired: 2 in, 2 out]
                    n105 = property on="System ind." class="DigNum (strict)"("Visible"=w186) -> ()  [unwired: 2 in, 2 out]
                    n106 = property on="RS232 Config. System" class="Clust (strict)"("Visible"=FALSE ("Write Attribute")) -> ()  [unwired: 2 in, 2 out]
                  }
                  frame 2 {
                    w188 = FALSE ("Write Attribute")
                    n107 = property on="GPIB Configuration system" class="Clust (strict)"("Visible"=w188) -> ()  [unwired: 2 in, 2 out]
                    n108 = property on="RS232 Config. System" class="Clust (strict)"("Visible"=w188) -> ()  [unwired: 2 in, 2 out]
                    n109 = property on="System ind." class="DigNum (strict)"("Visible"=w188) -> ()  [unwired: 2 in, 2 out]
                  }
                }
              }
              frame 3 {
                w190 = TRUE ("Write Attribute")
                w189 = FALSE ("Write Attribute")
                n110 = property on="System ind." class="DigNum (strict)"("Visible"=w190) -> ()  [unwired: 2 in, 2 out]
                n111 = property on="TCP/IP Config. System" class="Clust (strict)"("Visible"=w190) -> ()  [unwired: 2 in, 2 out]
                n112 = property on="GPIB Configuration system" class="Clust (strict)"("Visible"=w189) -> ()  [unwired: 2 in, 2 out]
                n113 = property on="RS232 Config. System" class="Clust (strict)"("Visible"=w189) -> ()  [unwired: 2 in, 2 out]
                n114 = property on="DLL for Device" class="Ring (strict)"("Visible"=w189) -> ()  [unwired: 2 in, 2 out]
              }
            }
            n115 = property on="Send" class="Str"("Key Focus"=TRUE ("Write Attribute")) -> ()  [unwired: 2 in, 2 out]
          }
          frame True {
            n116 = Add(x=w199, y=1) -> (x+y=w195:i32)
            n117 = local read "Send"() -> (w207:string)
            n118 = String Length(string=w207) -> (length=w201:i32)
            n119 = Subtract(x=w201, y=w196) -> (x-y=w206:i32)
            n120 = String Subset(string=w207, offset (0)=w196, length (rest)=w206) -> (substring=w202:string)
            n121 = call "Analyse input string for terminal.vi"("Last string sent"=w208, "String new"=w202) -> ("String out"=w205:string, "Out not equal to in?"=w203:bool, "Attach term. char.?"=w191:bool)  [unwired: 15 out]
            n122 = case shown="True" w203 {
              tunnel: w205 -> [w220 w226]
              tunnel: [w217 w224] -> w200
              tunnel: w204 -> [w223 w227]
              tunnel: w202 -> [w222 _]
              frame True {
                n123 = Concatenate Strings(w223, w222, "  (Sent: " ("Substring"), w220, ")" ("Substring"), "\n") -> (w217:string)
                n124 = local write "Send"(w217) -> ()
              }
              frame False {
                n125 = Concatenate Strings(w227, w226, "\n") -> (w224:string)
                n126 = local write "Send"(w224) -> ()
              }
            }
            n127 = stacked-sequence {
              tunnel: [w215] -> w197
              tunnel: w200 -> [w216]
              frame #0 {
                n128 = String Length(string=w216) -> (length=w215:i32)
                n129 = property on="Send" class="Str"("Text.Selection:Start"=w215, "Text.Selection:End"=w215) -> ()  [unwired: 2 in, 2 out]
              }
            }
            n130 = stacked-sequence {
              tunnel: w197 -> [w212]
              tunnel: [w212] -> w194
              tunnel: w195 -> [w211]
              frame #0 {
                n131 = property on="Send" class="Str"("Text.Scroll Position"=w211) -> ()  [unwired: 2 in, 2 out]
              }
            }
            n132 = call "PI Send String.vi"("System no."=w210, "String to send"=w205, "Attach termination char.?"=w191) -> ("error out"=w192:errorcluster)  [unwired: 1 in, 15 out]
            "error out" <- w192
            n133 = stacked-sequence {
              tunnel: w194 -> [w213]
              tunnel: [w213] -> w193
              tunnel: w192 -> [_]
              frame #0 {
                n134 = property on="Send" class="Str"("Key Focus"=TRUE ("Write Attribute")) -> ()  [unwired: 2 in, 2 out]
              }
            }
            n135 = Unbundle By Name(w192) -> ("status"=w209:bool)
            n136 = local write "error"(w209) -> ()
          }
        }
        n137 = case shown="False" "Clear" {
          tunnel: [w137 ""] -> w103
          tunnel: w106 -> [w137 _]
          tunnel: [w136 0] -> w104
          tunnel: w105 -> [w136 _]
          frame False {
          }
          frame True {
            n138 = local write "Receive"("") -> ()
          }
        }
        n139 = case shown="0, Default" "View style" {
          tunnel: [u32 0 ("Write Attribute") u32 1 ("Write Attribute") u32 3 ("Write Attribute")] -> w118
          frame 0, Default {
          }
          frame 1 {
          }
          frame 2 {
          }
        }
        n140 = stacked-sequence {
          tunnel: w115 -> [_]
          tunnel: w114 -> [w155]
          tunnel: [w154] -> w113
          tunnel: [w153] -> w111
          tunnel: w103 -> [_]
          frame #0 {
            n141 = call "PI Receive String.vi"("System no."=w155, "Strip spaces?"=FALSE) -> ("String read"=w153:string, "bytes read"=w154:u16)  [unwired: 1 in, 15 out]
          }
        }
        n142 = property on="Receive" class="Str"("Display Style"=w118) -> ()  [unwired: 2 in, 2 out]
        n143 = Greater?(x=w113, y=u16 1) -> (0:w102:bool)
        n144 = case shown="True" w102 {
          tunnel: [w142 w148] -> w101
          tunnel: w111 -> [_ w150]
          tunnel: w103 -> [w142 w151]
          tunnel: [w141 w146] -> w99
          tunnel: w104 -> [w141 w147]
          frame False {
          }
          frame True {
            n145 = Concatenate Strings(w151, w150, "\n" ("string")) -> (w148:string)
            n146 = call "How often does string contain regular expression?.vi"("Regular expression"="\\n" ("regular expression"), "String"=w150) -> ("Number"=w145:i32)  [unwired: 17 out]
            n147 = Increment(x=w145) -> (x+1=w143:i32)
            n148 = local write "Receive"(w148) -> ()
            n149 = Add(x=w143, y=w147) -> (x+y=w146:i32)
          }
        }
        n150 = case shown="True" "Show help" {
          frame False {
          }
          frame True {
            n151 = property on="Send" class="Str"("Visible"=FALSE ("Write Attribute")) -> ()  [unwired: 2 in, 2 out]
            n152 = property on="String" class="Str"("Visible"=TRUE ("Write Attribute")) -> ()  [unwired: 2 in, 2 out]
            n153 = while {
              tunnel: [w131] -> w128
              stop <- w131 continue-if-true
              n154 = Not(x="Hide help") -> (.not. x?=w131:bool)
            }
            n155 = Not(x=w128) -> (.not. x?=w127:bool)
            n156 = property on="Send" class="Str"("Visible"=w127) -> ()  [unwired: 2 in, 2 out]
            n157 = property on="String" class="Str"("Visible"=w128) -> ()  [unwired: 2 in, 2 out]
          }
        }
        n158 = case shown="False" w102 {
          tunnel: w101 -> [w133 w135]
          tunnel: [w133 w135] -> w100
          tunnel: w99 -> [_ w134]
          frame False {
          }
          frame True {
            n159 = property on="Receive" class="Str"("Text.Scroll Position"=w134) -> ()  [unwired: 2 in, 2 out]
          }
        }
        n160 = local read "Exit"() -> (w97:bool)
        n161 = Not(x=w97) -> (.not. x?=w96:bool)
        n162 = Wait Until Next ms Multiple(millisecond multiple=u32 10) -> ()  [unwired: 1 out]
      }
      n163 = property on="Send" class="Str"("Key Focus"=TRUE ("Write Attribute")) -> ()  [unwired: 2 in, 2 out]
      n164 = local write "Exit"(w81) -> ()
    }
    frame #3 {
      n165 = case shown="True" "ERR? on exit?" {
        tunnel: w235 -> [_ w267]
        tunnel: w234 -> [_ w266]
        tunnel: w233 -> [_ w265]
        tunnel: w232 -> [_ w264]
        tunnel: w231 -> [_ w263]
        tunnel: ["" w240] -> w228
        frame False {
        }
        frame True {
          n166 = local read "System No."() -> (w259:i32)
          n167 = Add(x=w265, y=1) -> (x+y=w255:i32)
          n168 = local read "Send"() -> (w250:string)
          n169 = String Length(string=w250) -> (length=w247:i32)
          n170 = Subtract(x=w247, y=w267) -> (x-y=w249:i32)
          n171 = String Subset(string=w250, offset (0)=w267, length (rest)=w249) -> (substring=w248:string)
          n172 = call "Analyse input string for terminal.vi"("Last string sent"="ERR?", "String new"=w248) -> ("String out"=w262:string)  [unwired: 17 out]
          n173 = Concatenate Strings(w266, w248, "  (Sent: " ("Substring"), w262, ")" ("Substring"), "\n") -> (w261:string)
          n174 = stacked-sequence {
            tunnel: [w273] -> w245
            tunnel: w261 -> [w274]
            frame #0 {
              n175 = String Length(string=w274) -> (length=w273:i32)
              n176 = property on="Send" class="Str"("Text.Selection:Start"=w273, "Text.Selection:End"=w273) -> ()  [unwired: 2 in, 2 out]
            }
          }
          n177 = stacked-sequence {
            tunnel: w245 -> [w270]
            tunnel: [w270] -> w244
            tunnel: w255 -> [w269]
            frame #0 {
              n178 = property on="Send" class="Str"("Text.Scroll Position"=w269) -> ()  [unwired: 2 in, 2 out]
            }
          }
          n179 = stacked-sequence {
            tunnel: w244 -> [w271]
            tunnel: [w271] -> w260
            frame #0 {
              n180 = property on="Send" class="Str"("Key Focus"=TRUE ("Write Attribute")) -> ()  [unwired: 2 in, 2 out]
            }
          }
          n181 = stacked-sequence {
            tunnel: w260 -> [_]
            tunnel: w259 -> [w289]
            tunnel: [w288] -> w258
            tunnel: [w287] -> w256
            tunnel: w264 -> [_]
            frame #0 {
              n182 = call "PI Receive String.vi"("System no."=w289) -> ("String read"=w287:string, "bytes read"=w288:u16)  [unwired: 2 in, 15 out]
            }
          }
          n183 = Greater?(x=w258, y=u16 1) -> (0:w254:bool)
          n184 = case shown="True" w254 {
            tunnel: [w279 w283] -> w253
            tunnel: w256 -> [_ w285]
            tunnel: w264 -> [w279 w286]
            tunnel: [w278 w280] -> w252
            tunnel: w263 -> [w278 w281]
            frame False {
            }
            frame True {
              n185 = Concatenate Strings(w286, w285) -> (w283:string)
              n186 = call "How often does string contain regular expression?.vi"("Regular expression"="\\n" ("regular expression"), "String"=w285) -> ("Number"=w282:i32)  [unwired: 17 out]
              n187 = local write "Receive"(w283) -> ()
              n188 = Add(x=w282, y=w281) -> (x+y=w280:i32)
            }
          }
          n189 = local write "Send"(w261) -> ()
          n190 = call "PI Send String.vi"("System no."=w259, "String to send"=w262, "Attach termination char.?"=TRUE ("Attach Linefeed?")) -> ()  [unwired: 1 in, 16 out]
          n191 = case shown="True" w254 {
            tunnel: w253 -> [w275 w277]
            tunnel: [w275 w277] -> w240
            tunnel: w252 -> [_ w276]
            frame False {
            }
            frame True {
              n192 = property on="Receive" class="Str"("Text.Scroll Position"=w276) -> ()  [unwired: 2 in, 2 out]
            }
          }
        }
      }
      n193 = for {
        N: w229 -> [_]
        tunnel: w228 -> [_]
        i -> [w238]
        n194 = Increment(x=w238) -> (x+1=w237:i32)
        n195 = call "Close connection if open.vi"("System no."=w237, "Close DaisyChain"=TRUE) -> ()  [unwired: 1 in, 17 out]
      }
    }
  }
